vi "load cDAQ settings.vi"() -> (3 "cDAQ Settings":T1)   [LabVIEW 2014]
uses:
  TypeDef/cDAQ Settings.ctl
  <vilib>/Utility/file.llb/Read From Spreadsheet File (string).vi
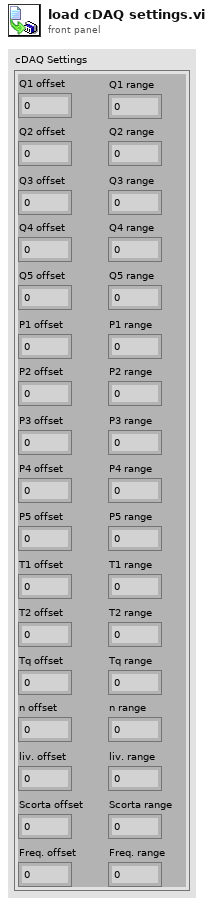
[diagram p1: front panel]
types:
  T1 = typedef "cDAQ Settings.ctl" = cluster{"Q1 offset":dbl, "Q1 range":dbl, "Q2 offset":dbl, "Q2 range":dbl, "Q3 offset":dbl, "Q3 range":dbl, "P3 offset":dbl, "P3 range":dbl, "P4 offset":dbl, "P4 range":dbl, "liv. offset":dbl, "liv. range":dbl, "Scorta offset":dbl, "Scorta range":dbl, "Freq. offset":dbl, "Freq. range":dbl, "Q4 range":dbl, "Q4 offset":dbl, "Q5 range":dbl, "Q5 offset":dbl, "P1 range":dbl, "P1 offset":dbl, "P2 range":dbl, "P2 offset":dbl, "P5 range":dbl, "P5 offset":dbl, "T1 range":dbl, "T1 offset":dbl, "T2 range":dbl, "T2 offset":dbl, "Tq range":dbl, "Tq offset":dbl, "n range":dbl, "n offset":dbl}
  T2 = cluster{"[0]":dbl, "[1]":dbl, "[2]":dbl, "[3]":dbl, "[4]":dbl, "[5]":dbl, "[6]":dbl, "[7]":dbl, "[8]":dbl, "[9]":dbl, "[10]":dbl, "[11]":dbl, "[12]":dbl, "[13]":dbl, "[14]":dbl, "[15]":dbl, "[16]":dbl, "[17]":dbl, "[18]":dbl, "[19]":dbl, "[20]":dbl, "[21]":dbl, "[22]":dbl, "[23]":dbl, "[24]":dbl, "[25]":dbl, "[26]":dbl, "[27]":dbl, "[28]":dbl, "[29]":dbl, "[30]":dbl, "[31]":dbl, "[32]":dbl, "[33]":dbl}
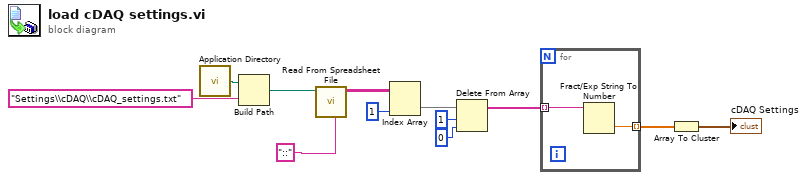
[diagram p0: block diagram]
diagram:
  n1 = call <vilib>:"Application Directory.vi"() -> ("Application Directory"=w12:path)
  n2 = Build Path(base path=w12, name or relative path="Settings\\cDAQ\\cDAQ_settings.txt") -> (appended path=w10:path)
  n3 = call-poly <vilib>:"Read From Spreadsheet File.vi"("delimiter (\\t)"="::" ("delimiter (\\t)"), "file path (dialog if empty)"=w10) -> ("all rows"=w8:string[][])  [unwired: 5 in, 4 out]
  n4 = Index Array(array=w8, index (col)=1 ("disabled index (col)")) -> (element=w5:string[])  [unwired: 1 in]
  n5 = Delete From Array(array=w5, length=1, index=0) -> (array with subset deleted=w2:string[])  [unwired: 1 out]
  n6 = for {
    tunnel: w2 -> [w14] mode=indexing
    tunnel: [w13] -> w6 mode=indexing
    n7 = Fract/Exp String To Number(string=w14) -> (number=w13:dbl)  [unwired: 3 in, 1 out]
  }
  n8 = Array To Cluster(array=w6) -> (cluster=→"cDAQ Settings":T2)
